vi "Launcher.vi"() -> ()   [LabVIEW 2020]
uses:
  UI Actor/UI Actor.lvclass
  C:/Program Files (x86)/National Instruments/LabVIEW 2020/vi.lib/ActorFramework/Actor/Actor.lvclass
  UI Actor/UI Actor.lvclass/UI Actor.ctl
  UI Actor/Write Coins.vi
  UI Actor/Write Productos.vi
  UI Actor/Write Msg.vi
  <vilib>/ActorFramework/Actor/Actor.lvclass
panel:
  in  "Msg":enum16{"Español", "English"}(ring)
  in  "Productos":enum16{"Nestle", "Coca"}(ring)
  in  "Coins":enum16{"MX", "USD"}(ring)
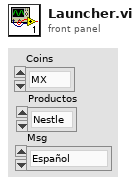
[diagram p1: front panel]
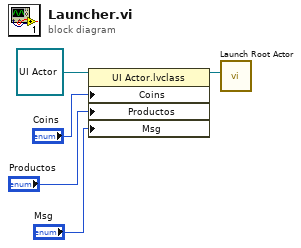
[diagram p0: block diagram]
diagram:
  n1 = property class="UI Actor.lvclass"(reference=refnum<class "UI Actor.lvclass"> refnum ("UI Actor.lvlib:UI Actor.lvclass"), "Coins"="Coins", "Productos"="Productos", "Msg"="Msg") -> (reference out=w4:refnum<class "UI Actor.lvclass">)  [unwired: 1 in, 1 out]
  n2 = call <vilib>:"Launch Root Actor.vi"("Actor"=w4) -> ()  [unwired: 9 in, 2 out]
